vi "Help_Prompt-W.vi"(2 "error in (no error)":errorcluster, 3 "Data Cluster":T1 {"Shaft"."dmin" format="%#_7g"; "Shaft"."dmax" format="%#_7g"; "Shaft"."Fundamental Dev" format="%#_7g"; "Shaft"."Tolerance Grade (IT) Shaft" format="%#_7g"; "Hole"."Dmin" format="%#_7g"; "Hole"."Tolerance Grade (IT)" format="%#_7g"}, 4 "Panel In":refnum<class "Panel.lvclass">) -> (0 "error out":errorcluster)   [LabVIEW 2023]
uses:
  TypeDef/Help_Menu.ctl
  <vilib>/MGI/Panel Manager/Panel/Panel/Panel.lvclass
  TypeDef/Data_Cluster.ctl
  TypeDef/Units.ctl
  TypeDef/Method_Info.ctl
  TypeDef/Hole_Data.ctl
  TypeDef/Shaft_Data.ctl
  <userlib>/_OpenG.lib/appcontrol/appcontrol.llb/openg_application_control.lvlib
panel:
  out "Information":string
  in  "Help Menu":T6
  in  "Close Button":bool
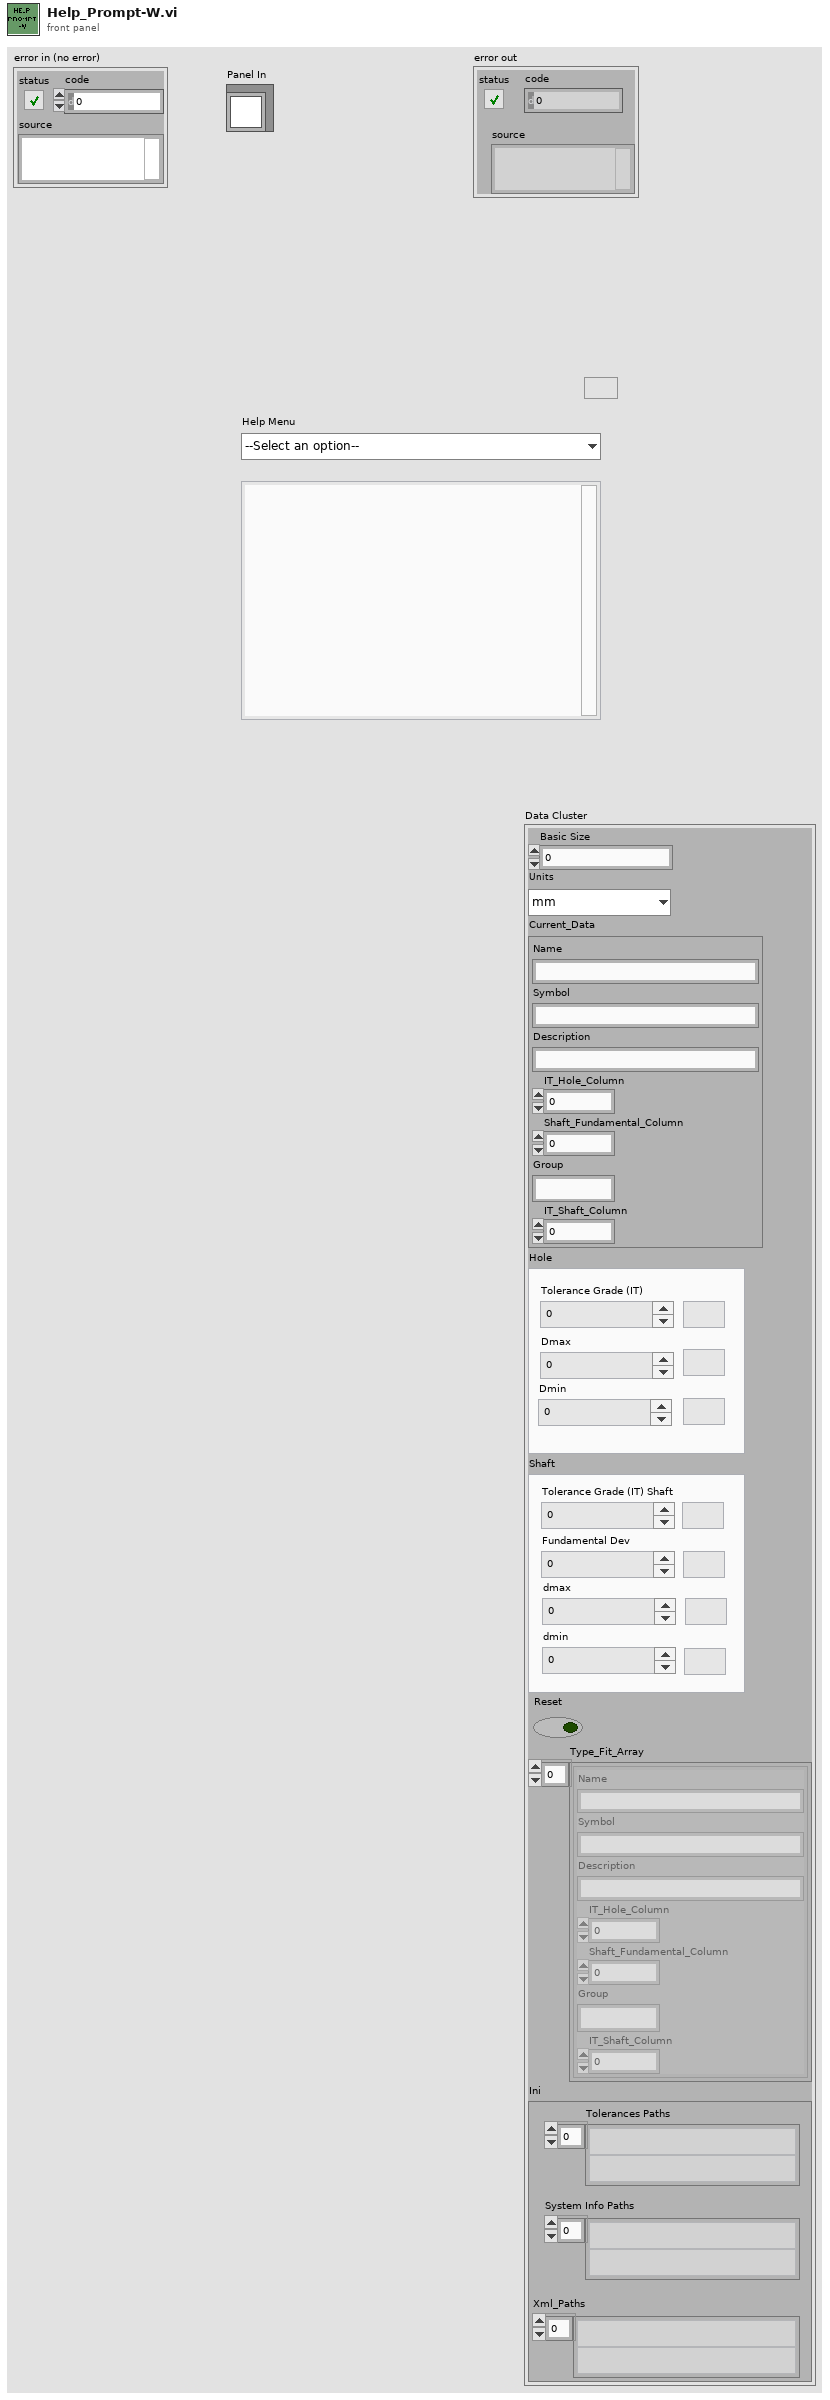
[diagram p1: front panel]
types:
  T1 = typedef "Data_Cluster.ctl" = cluster{"Basic Size ":dbl, "Units":T2, "Current_Data":T3, "Hole":T4, "Shaft":T5, "Reset":bool, "Type_Fit_Array":T3[], "Ini":cluster{"Tolerances Paths":path[], "System Info Paths":path[], "Xml_Paths":path[]}}
  T2 = typedef "Units.ctl" = enum16{"mm", "in"}
  T3 = typedef "Method_Info.ctl" = cluster{"Name":string, "Symbol":string, "Description":string, "IT_Hole_Column":i32, "Shaft_Fundamental_Column":i32, "Group":string, "IT_Shaft_Column":i32}
  T4 = typedef "Hole_Data.ctl" = cluster{"Tolerance Grade (IT)":dbl, "Dmax":dbl, "Units Hole":cluster{"units_it":string, "units_Dmax\nUnits_Dmax":string, "Units_Dmin":string}, "Dmin":dbl}
  T5 = typedef "Shaft_Data.ctl" = cluster{"Tolerance Grade (IT) Shaft":dbl, "Units Shaft":cluster{"Units_FundamentalDev":string, "Units_dmax":string, "Units_dmin":string, "Units_IT_Shaft":string}, "Fundamental Dev":dbl, "dmax":dbl, "dmin":dbl}
  T6 = typedef "Help_Menu.ctl" = enum16{"--Select an option--", "Basic concepts", "Drawing", "References", "Support"}
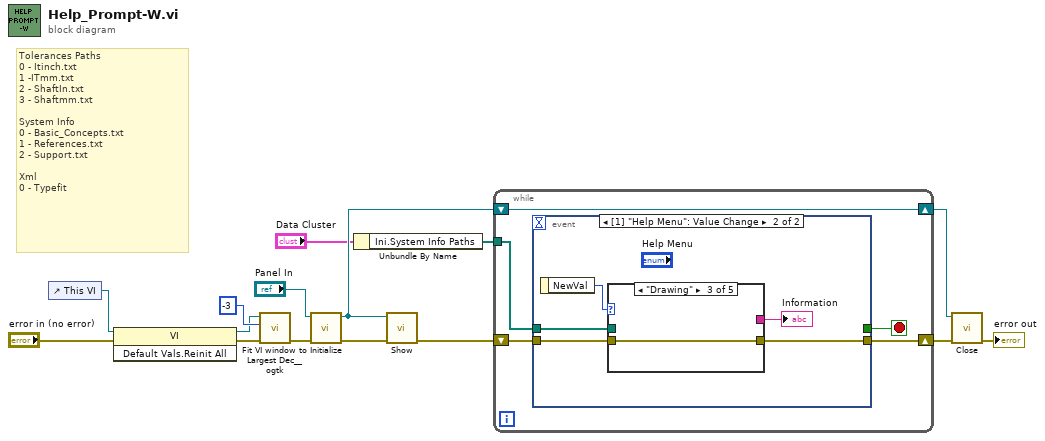
[diagram p0: block diagram]
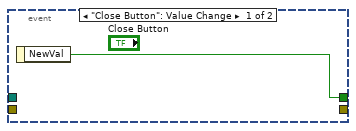
[diagram p2: hidden frame]
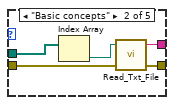
[diagram p4: hidden frame]
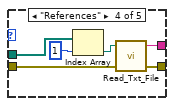
[diagram p5: hidden frame]
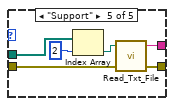
[diagram p6: hidden frame]
diagram:
  # "Tolerances Paths\n0 - Itinch.txt\n1 -ITmm.txt\n2 - ShaftIn.txt\n3 - Shaftmm.txt\n\nSystem Info \n0 - Basic_Concepts.txt\n1 - References.txt\n2 - Support.txt\n\nXml\n0 - Typefit"
  n1 = control-ref of="This VI"() -> (w6:refnum<vi>)
  n2 = invoke class="VI" method="Default Vals.Reinit All"(reference=w6, error in="error in (no error)") -> (reference out=w4:refnum<vi>, error out=w5:errorcluster)  [unwired: 1 in, 1 out]
  n3 = call <userlib>:"Fit VI window to Largest Dec__ogtk.vi"("error in (no error)"=w5, "border spacing (2 px)"=-3, "VI Ref (calling VI)"=w4) -> ("error out"=w12:errorcluster)  [unwired: 3 in, 1 out]
  n4 = call <vilib>:"Initialize.vi"("error in (no error)"=w12, "Panel In"="Panel In") -> ("error out"=w11:errorcluster, "Panel Out"=w7:refnum<class "Panel.lvclass">)  [unwired: 7 in, 1 out]
  n5 = Unbundle By Name("Data Cluster") -> ("Ini.System Info Paths"=w1:path[])
  n6 = call <vilib>:"Show.vi"("Error In"=w11, "Panel in"=w7) -> ("Error Out"=w8:errorcluster)  [unwired: 9 in]
  n7 = while {
    shift-right: [w18] -> w14
    shift-left: w8 -> [w19]
    shift-right: [w17] -> w10
    shift-left: w7 -> [w17]
    tunnel: w1 -> [w16]
    stop <- w20 stop-if-true
    n8 = event shown="[1] \"Help Menu\": Value Change" {
      selector: _ -> [_ _]
      dyn-events: _ -> [_ _]
      timeout: _ -> [_ _]
      tunnel: [w21 _] -> w20
      tunnel: w19 -> [_ w26]
      tunnel: [_ w25] -> w18
      tunnel: w16 -> [_ w23]
      event "Close Button": Value Change {
        n9 = event-data() -> ("NewVal"=w21:bool)  [unwired: 1 in]
      }
      event Value Change {
        n10 = event-data() -> ("NewVal"=w24:T6)  [unwired: 1 in]
        n11 = case shown="\"Drawing\"" w24 {
          tunnel: w26 -> [w27 w32 w33 w38 w40]
          tunnel: [w27 w31 w33 w39 w42] -> w25
          tunnel: w23 -> [_ w29 _ w37 w45]
          tunnel: [_ w30 _ w35 w41] -> w22
          frame "--Select an option--", Default {
          }
          frame "Basic concepts" {
            n12 = Index Array(array=w29) -> (element=w28:path)  [unwired: 1 in]
            n13 = call "Read_Txt_File.vi"("error in (no error)"=w32, "Path"=w28) -> ("error out"=w31:errorcluster, "Text"=w30:string)  [unwired: 2 in]
          }
          frame "Drawing" {
          }
          frame "References" {
            n14 = Index Array(array=w37, index=1) -> (element=w36:path)
            n15 = call "Read_Txt_File.vi"("error in (no error)"=w38, "Path"=w36) -> ("error out"=w39:errorcluster, "Text"=w35:string)  [unwired: 2 in]
          }
          frame "Support" {
            n16 = Index Array(array=w45, index=2) -> (element=w43:path)
            n17 = call "Read_Txt_File.vi"("error in (no error)"=w40, "Path"=w43) -> ("error out"=w42:errorcluster, "Text"=w41:string)  [unwired: 2 in]
          }
        }
        "Information" <- w22
      }
    }
  }
  n18 = call-dynamic "Close.vi"("Error In"=w14, "Panel In"=w10) -> ("Error Out"=→"error out":errorcluster)  [unwired: 9 in]
